vi "MT Add MultiTone.vi"(0 "input complex waveform":T1={"t0"=0.0, "dt"=1.0, "Y"=[]} {"Y" format="%.3f"; "dt" format="%^.2e"; "t0" format="%.4f"}, 5 "tones":cluster{"freq (Hz)":dbl, "amplitude (dB)":dbl}[](array[cluster]) {"amplitude (dB)" format="%.2f"; "freq (Hz)" format="%.2f"}, 9 "reference power (dBm)":dbl format="%.2f", 11 "error in (no error)":errorcluster, 13 "reset? (T)":bool=TRUE) -> (4 "output complex waveform":T1 {"Y" format="%.3f"; "dt" format="%^.2e"; "t0" format="%.4f"}, 15 "error out":errorcluster)   [LabVIEW 2020, in "niDMT.lvlib"]
doc: "Generates a multitone waveform, adds it to the complex baseband modulated waveform, and returns a signal-plus-tones waveform. You can use the tones-added signal to test transmitter interference rejection."
uses:
  <vilib>/addons/Modulation/niDMT.lvlib
  <vilib>/addons/Modulation/Analog/controls/Complex Data Waveform.ctl
  <vilib>/addons/Modulation/niAMT.lvlib
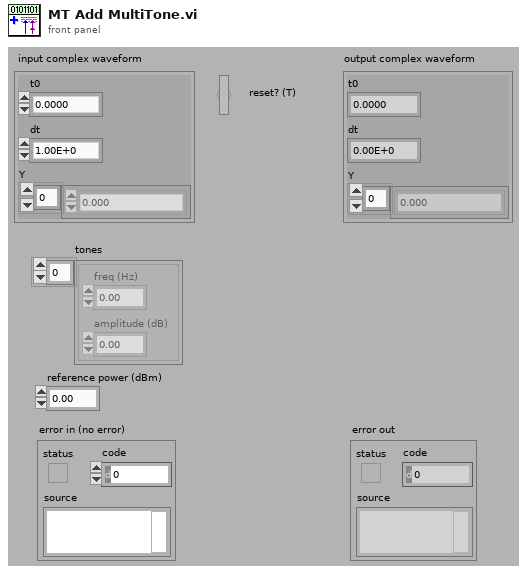
[diagram p1: front panel]
types:
  T1 = typedef "niAMT.lvlib/Complex Data Waveform.ctl" = cluster{"t0":dbl, "dt":dbl, "Y":cdb[]}
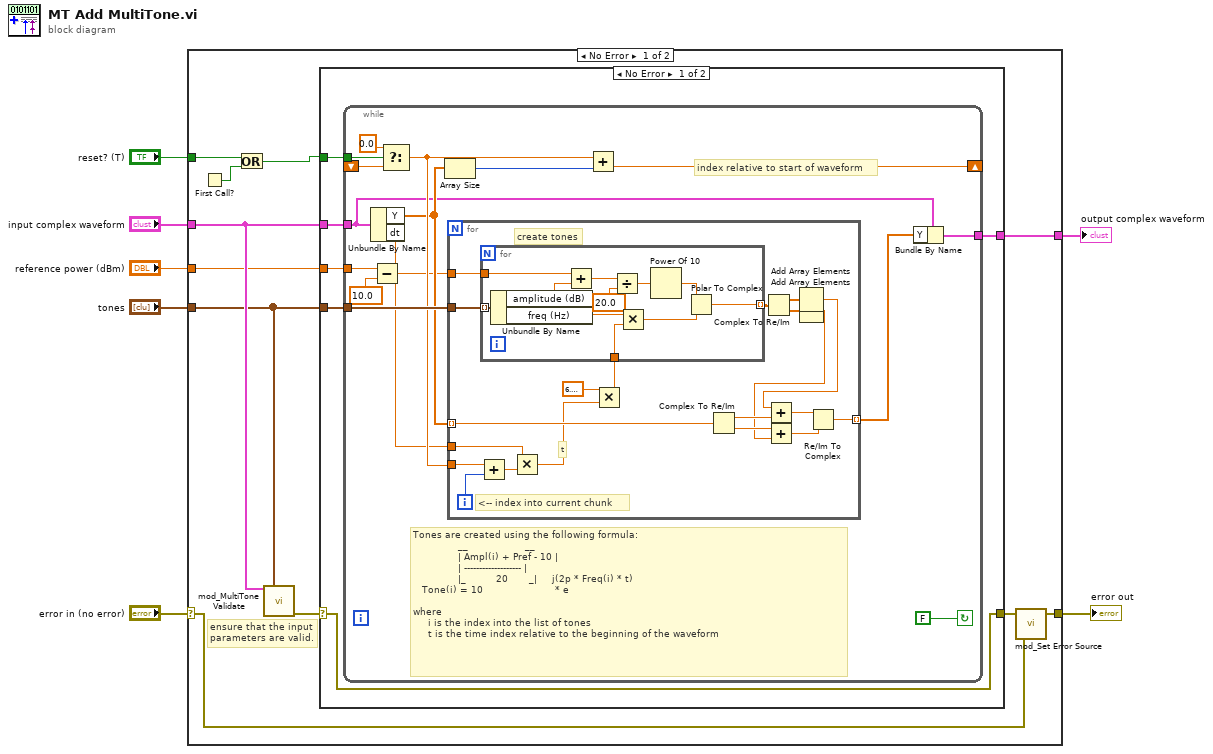
[diagram p0: block diagram]
diagram:
  n1 = case shown="No Error" "error in (no error)" {
    selector: "error in (no error)" -> [w11 w73]
    tunnel: [w13 w73] -> w6
    tunnel: "input complex waveform" -> [w17 _]
    tunnel: "tones" -> [w16 _]
    tunnel: "reference power (dBm)" -> [w15 _]
    tunnel: "reset? (T)" -> [w10 _]
    tunnel: [w14 _] -> w1
    frame No Error {
      # "ensure that the input parameters are valid."
      n2 = First Call?() -> (First Call?: T/F=w9:bool)
      n3 = Or(x=w10, y=w9) -> (x .or. y?=w8:bool)
      n4 = call <vilib>:"mod_MultiTone Validate.vi"("Input Complex Waveform"=w17, "Tones"=w16) -> ("error out"=w18:errorcluster)  [unwired: 1 in, 12 out]
      n5 = case shown="No Error" w18 {
        selector: w18 -> [w19 w72]
        tunnel: [w19 w72] -> w12
        tunnel: w8 -> [w24 _]
        tunnel: w17 -> [w23 _]
        tunnel: w16 -> [w22 _]
        tunnel: w15 -> [w21 _]
        tunnel: [w20 _] -> w14
        frame No Error {
          n6 = while {
            shift-right: [w32] -> _
            shift-left: _ -> [w40]
            tunnel: w24 -> [w38]
            tunnel: w23 -> [w31]
            tunnel: w22 -> [w36]
            tunnel: w21 -> [w27]
            tunnel: [w29] -> w20
            stop <- FALSE continue-if-true
            # "Tones are created using the following formula:\n               __                   __ \n               | Ampl(i) + Pref - 10 |\n               | ------------------- |\n               |_          20       _|     j(2p * Freq(i) * t)\n   Tone(i) = 10                        * e\n\nwhere \n     i is the index into the list of tones\n     t is the time index relative to the beginning of the waveform"
            # "index relative to start of waveform"
            n7 = Unbundle By Name(w31) -> ("Y"=w33:cdb[], "dt"=w34:dbl)
            n8 = Subtract(x=w27, y=10.0) -> (x-y=w25:dbl)
            n9 = Select(t=0.0, s=w38, f=w40) -> (s? t:f=w35:dbl)
            n10 = Array Size(array=w33) -> (size(s)=w37:i32)
            n11 = for {
              tunnel: w36 -> [w60]
              tunnel: w35 -> [w58]
              tunnel: w34 -> [w56]
              tunnel: w33 -> [w55] mode=indexing
              tunnel: [w50] -> w30 mode=indexing
              tunnel: w25 -> [w41]
              i -> [w59]
              # "t"
              # "<-- index into current chunk"
              # "create tones"
              n12 = Add(x=w58, y=w59) -> (x+y=w57:dbl)
              n13 = Multiply(x=w56, y=w57) -> (x*y=w44:dbl)
              n14 = Multiply(x=6.283185307179586, y=w44) -> (x*y=w42:dbl)
              n15 = for {
                tunnel: w60 -> [w71] mode=indexing
                tunnel: [w65] -> w47 mode=indexing
                tunnel: w42 -> [w63]
                tunnel: w41 -> [w61]
                n16 = Unbundle By Name(w71) -> ("amplitude (dB)"=w70:dbl, "freq (Hz)"=w64:dbl)
                n17 = Add(x=w61, y=w70) -> (x+y=w69:dbl)
                n18 = Divide(x=w69, y=20.0) -> (x/y=w67:dbl)
                n19 = Multiply(x=w64, y=w63) -> (x*y=w62:dbl)
                n20 = Power Of 10(x=w67) -> (10^x=w66:dbl)
                n21 = Polar To Complex(1:w62, 2:w66) -> (0:w65:cdb)
              }
              n22 = Complex To Re/Im(x + iy=w55) -> (x=w54:dbl, y=w53:dbl)
              n23 = Complex To Re/Im(x + iy=w47) -> (x=w46:dbl[], y=w45:dbl[])
              n24 = Add Array Elements(numeric array=w46) -> (sum=w49:dbl)
              n25 = Add(x=w49, y=w54) -> (x+y=w52:dbl)
              n26 = Add Array Elements(numeric array=w45) -> (sum=w48:dbl)
              n27 = Add(x=w53, y=w48) -> (x+y=w51:dbl)
              n28 = Re/Im To Complex(1:w51, 2:w52) -> (0:w50:cdb)
            }
            n29 = Add(x=w35, y=w37) -> (x+y=w32:dbl)
            n30 = Bundle By Name(cluster=w31, "Y"=w30) -> (w29:T1)
          }
        }
        frame Error {
        }
      }
      n31 = call <vilib>:"mod_Set Error Source.vi"("initial error in (no error)"=w11, "final error in (no error)"=w12) -> ("error out"=w13:errorcluster)  [unwired: 1 in, 2 out]
    }
    frame Error {
    }
  }
  "error out" <- w6
  "output complex waveform" <- w1
